vi "Compare 1D Arrays - string.vi"(2 "New Array":string[](array[string]), 3 "Old Array":string[](array[string])) -> (0 "Removed":string[](array[string]), 1 "Added":string[](array[string]))   [LabVIEW 2013, in "FA_FIRST.lvlib"]
uses:
  FA_FIRST.lvlib
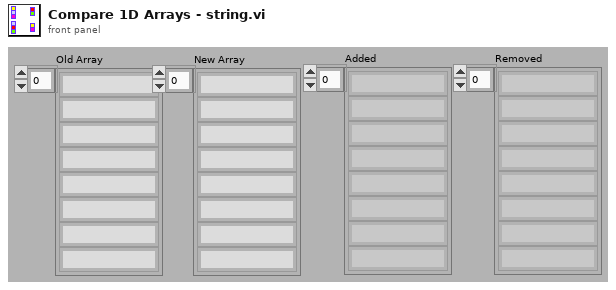
[diagram p1: front panel]
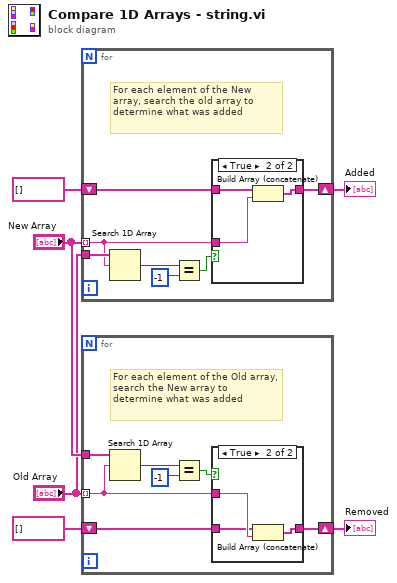
[diagram p0: block diagram]
diagram:
  n1 = for {
    tunnel: "New Array" -> [w9] mode=indexing
    tunnel: "Old Array" -> [w13]
    shift-right: [w8] -> w5
    shift-left: string[] [] -> [w7]
    # "For each element of the New array, search the old array to determine what was added"
    n2 = Search 1D Array(1D array=w13, element=w9) -> (index of element=w12:i32)  [unwired: 1 in]
    n3 = Equal?(x=w12, y=-1) -> (x = y?=w10:bool)
    n4 = case shown="True" w10 {
      tunnel: w9 -> [_ w17]
      tunnel: [w14 w16] -> w8
      tunnel: w7 -> [w14 w15]
      frame False {
      }
      frame True {
        n5 = Build Array (concatenate)(w15, w17) -> (w16:string[])
      }
    }
  }
  "Added" <- w5
  n6 = for {
    tunnel: "Old Array" -> [w20] mode=indexing
    tunnel: "New Array" -> [w24]
    shift-right: [w19] -> w2
    shift-left: string[] [] -> [w18]
    # "For each element of the Old array, search the New array to determine what was added"
    n7 = Search 1D Array(1D array=w24, element=w20) -> (index of element=w23:i32)  [unwired: 1 in]
    n8 = Equal?(x=w23, y=-1) -> (x = y?=w21:bool)
    n9 = case shown="True" w21 {
      tunnel: w20 -> [_ w28]
      tunnel: [w25 w27] -> w19
      tunnel: w18 -> [w25 w26]
      frame False {
      }
      frame True {
        n10 = Build Array (concatenate)(w26, w28) -> (w27:string[])
      }
    }
  }
  "Removed" <- w2
